vi "fattoriale.vi"(1 "n":u8=1 min=1 step=1) -> (0 "n!":dbl)   [LabVIEW 2021]
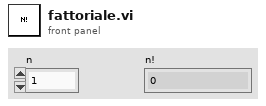
[diagram p1: front panel]
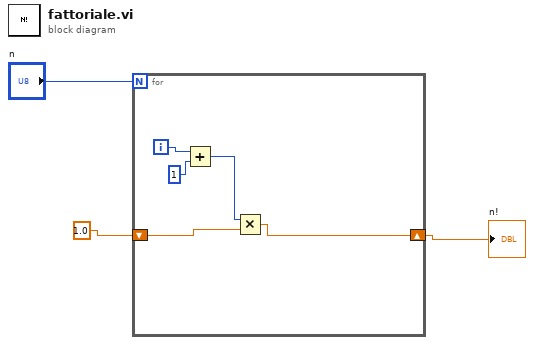
[diagram p0: block diagram]
diagram:
  n1 = for {
    N: "n" -> [_]
    shift-right: [w4] -> w1
    shift-left: 1.0 -> [w5]
    i -> [w8]
    n2 = Add(x=w8, y=1) -> (x+y=w6:i32)
    n3 = Multiply(x=w6, y=w5) -> (x*y=w4:dbl)
  }
  "n!" <- w1
